vi "Sub Str to hex array.vi"(1 "hex str":string) -> (0 "Hex array":u8[](array[numeric]))   [LabVIEW 2009]
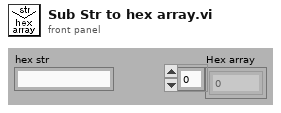
[diagram p1: front panel]
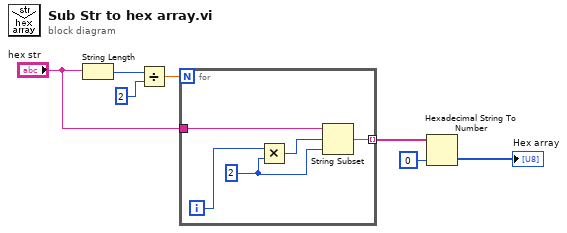
[diagram p0: block diagram]
diagram:
  n1 = String Length(string="hex str") -> (length=w1:i32)
  n2 = Divide(x=w1, y=2) -> (x/y=w3:dbl)
  n3 = for {
    N: w3 -> [_]
    tunnel: "hex str" -> [w12]
    tunnel: [w8] -> w4 mode=indexing
    i -> [w10]
    w9 = 2 ("길이(나머지)")
    n4 = Multiply(x=w10, y=w9) -> (x*y=w11:i32)
    n5 = String Subset(string=w12, offset (0)=w11, length (rest)=w9) -> (substring=w8:string)
  }
  n6 = Hexadecimal String To Number(string=w4, default (0uL)=u8 0 ("기본(0 U32)")) -> (number=→"Hex array":u8[])  [unwired: 1 in, 1 out]
